vi "publish -- num -- Real -- V2.vi"(7 "publisher action":T1, 10 "Numeric":dbl format="%#_13g") -> (0 "time out":timestamp, 2 "Numeric out":dbl)   [LabVIEW 2018]
uses:
  publisher action.ctl
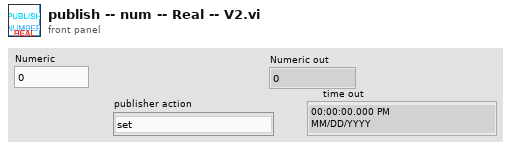
[diagram p1: front panel]
types:
  T1 = typedef "publisher action.ctl" = enum16{"set", "get", "init", "check"}
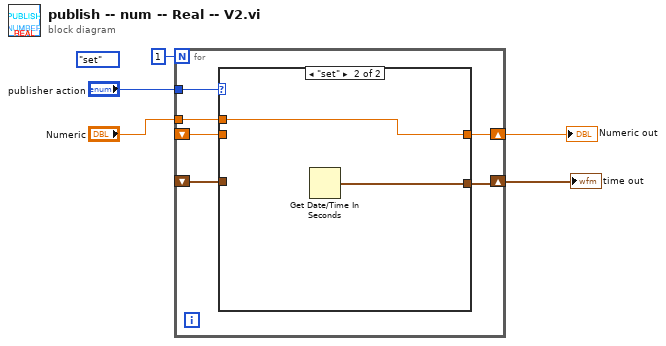
[diagram p0: block diagram]
diagram:
  (unwired) publisher_action."set" ("publisher action")
  n1 = for {
    N: 1 -> [_]
    shift-right: [w11] -> w2
    shift-left: _ -> [w9]
    tunnel: "publisher action" -> [w10]
    tunnel: "Numeric" -> [w8]
    shift-right: [w7] -> w1
    shift-left: _ -> [w6]
    n2 = case shown="\"set\"" w10 {
      tunnel: [w13 w15] -> w11
      tunnel: w9 -> [w13 _]
      tunnel: w8 -> [_ w15]
      tunnel: [w12 w14] -> w7
      tunnel: w6 -> [w12 _]
      frame "get", Default {
      }
      frame "set" {
        n3 = Get Date/Time In Seconds() -> (seconds since 1Jan1904=w14:timestamp)
      }
    }
  }
  "Numeric out" <- w2
  "time out" <- w1
